vi "Exercises_4-5.vi"(1 "Power":bool) -> ()   [LabVIEW 2014]
doc: "This VI simulates measuring a temperature using the temperature sensor on the DAQ Signal Accessory.\n\nIf you have a DAQ board or a DAQ Signal Accessory, then use the Thermometer VI instead."
uses:
  Control 1.ctl
panel:
  out "Temperature History":T1
  # "ON\n\nOFF"
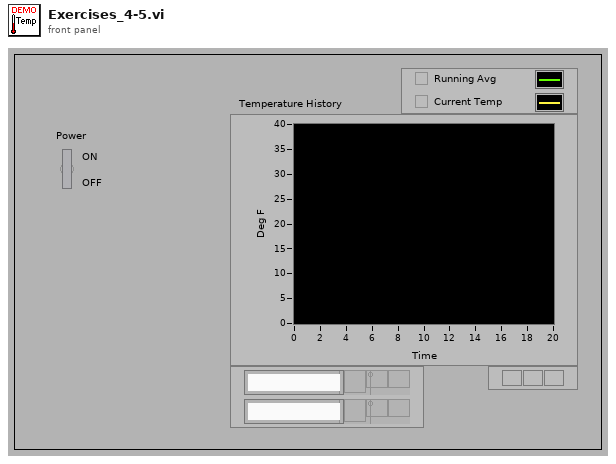
[diagram p1: front panel]
types:
  T1 = typedef "Control 1.ctl" = cluster{dbl, dbl}
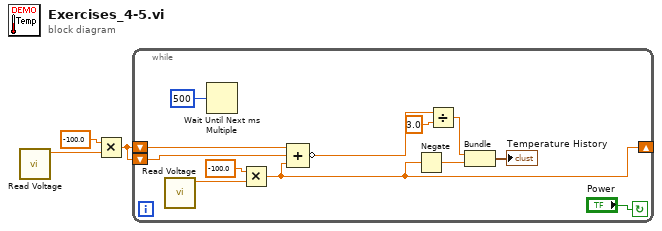
[diagram p0: block diagram]
diagram:
  n1 = call "Read Voltage.vi"() -> ("voltaje"=w2:dbl)  [unwired: 6 in, 1 out]
  n2 = Multiply(x=-100.0, y=w2) -> (x*y=w1:dbl)
  n3 = while {
    shift-right: [w4] -> _
    shift-left: w1 -> [w11]
    shift-left: w1 -> [w10]
    stop <- "Power" continue-if-true
    n4 = call "Read Voltage.vi"() -> ("voltaje"=w8:dbl)  [unwired: 6 in, 1 out]
    n5 = Wait Until Next ms Multiple(millisecond multiple=500) -> ()  [unwired: 1 out]
    n6 = Multiply(x=-100.0, y=w8) -> (x*y=w4:dbl)
    n7 = Compound Arithmetic op=ADD(w11, w10, w4) -> (invert w14:dbl)
    n8 = Negate(x=w4) -> (-x=w6:dbl)
    n9 = Divide(x=w14, y=3.0) -> (x/y=w7:dbl)
    n10 = Bundle(w7, w6) -> (→"Temperature History":cluster{dbl, dbl})  [unwired: 1 in]
  }
